vi "gsp_simulator_parse_command.vi"(4 "error in (no error)":errorcluster, 6 "commandstring":string) -> (0 "error out":errorcluster, 1 "Parameters":i32[](array[numeric]), 2 "Motor#":u8, 3 "Command#":u16)   [LabVIEW 2015]
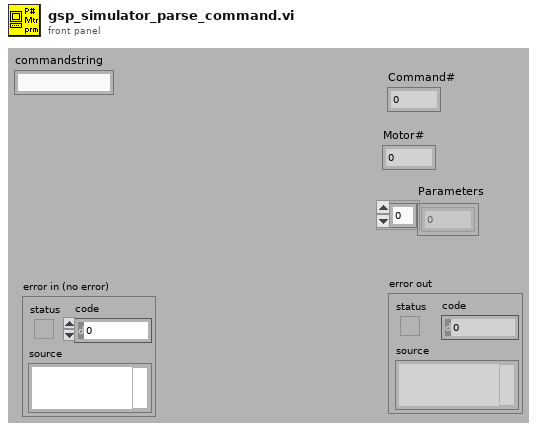
[diagram p1: front panel]
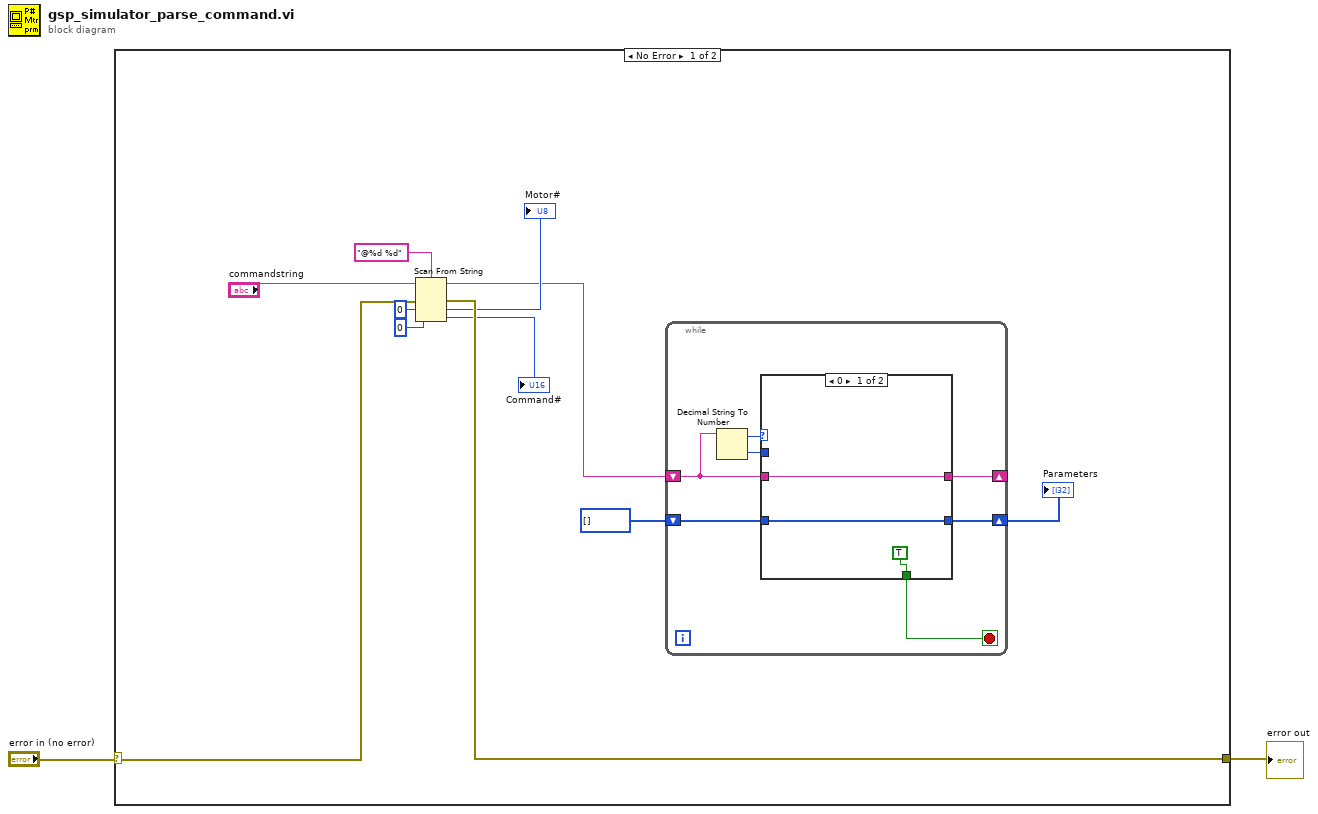
[diagram p0: block diagram]
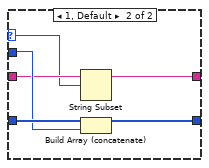
[diagram p2: hidden frame]
diagram:
  n1 = case shown="No Error" "error in (no error)" {
    selector: "error in (no error)" -> [w13 w30]
    tunnel: [w12 w30] -> w1
    frame No Error {
      n2 = Scan From String(format string="@%d %d", input string="commandstring", error in=w13, default 1=u8 0 ("default value 1"), default 2=u16 0 ("default value 2")) -> (remaining string=w5:string, error out=w12:errorcluster, output 1=→"Motor#":u8, output 2=→"Command#":u16)  [unwired: 1 in, 1 out]
      n3 = while {
        shift-right: [w15] -> w4
        shift-left: i32[] [] -> [w20]
        shift-right: [w14] -> _
        shift-left: w5 -> [w18]
        stop <- w17 stop-if-true
        n4 = Decimal String To Number(string=w18) -> (offset past number=w19:i32, number=w16:i32)  [unwired: 2 in]
        n5 = case shown="0" w19 {
          selector: w19 -> [_ w25]
          tunnel: w20 -> [w21 w29]
          tunnel: w18 -> [w22 w26]
          tunnel: [TRUE _] -> w17
          tunnel: w16 -> [_ w28]
          tunnel: [w21 w27] -> w15
          tunnel: [w22 w24] -> w14
          frame 0 {
          }
          frame 1, Default {
            n6 = String Subset(string=w26, offset (0)=w25) -> (substring=w24:string)  [unwired: 1 in]
            n7 = Build Array (concatenate)(w29, w28) -> (w27:i32[])
          }
        }
      }
      "Parameters" <- w4
    }
    frame Error {
    }
  }
  "error out" <- w1
